vi "Read LNA.vi"(8 "Error In":errorcluster, 11 "TestLNA in":refnum<class "TestLNA.lvclass">) -> (0 "Error Out":errorcluster, 2 "LNA Message Enqueuer":refnum<class "Message Enqueuer.lvclass">, 3 "TestLNA out":refnum<class "TestLNA.lvclass">)   [LabVIEW 2014, in "TestLNA.lvlib" / "TestLNA.lvclass"]
doc: "Read LNA enqueuer."
uses:
  TestLNA.lvclass
  <vilib>/ActorFramework/Message Enqueuer/Message Enqueuer.lvclass
  TestLNA.lvclass/TestLNA.ctl
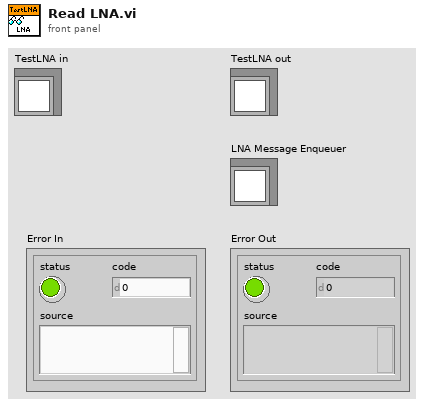
[diagram p1: front panel]
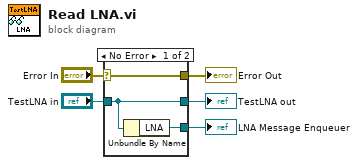
[diagram p0: block diagram]
diagram:
  n1 = case shown="No Error" "Error In" {
    selector: "Error In" -> [w8 w9]
    tunnel: [w8 w9] -> w4
    tunnel: [w7 w10] -> w2
    tunnel: "TestLNA in" -> [w7 w10]
    tunnel: [w6 _] -> w1
    frame No Error {
      n2 = Unbundle By Name(w7) -> ("LNA"=w6:refnum<class "Message Enqueuer.lvclass">)
    }
    frame Error {
    }
  }
  "Error Out" <- w4
  "TestLNA out" <- w2
  "LNA Message Enqueuer" <- w1
